vi "Numeric Speed to Formatted String.vi"(8 "error in (no error)":errorcluster, 9 "Speed Units":T1, 10 "Speed":dbl format="%.2f", 11 "ESM303 in":refnum<class "ESM303.lvclass">) -> (0 "error out":errorcluster, 2 "Formatted Speed String":string, 3 "ESM303 out":refnum<class "ESM303.lvclass">)   [LabVIEW 2018, in "ESM303.lvlib" / "ESM303.lvclass"]
uses:
  ESM303.lvclass
  builds/Force Test Stand/Force Test Stand/Force Test Stand.lvlibp/Custom Controls/Speed Units.ctl
  builds/Force Test Stand/Force Test Stand/Force Test Stand.lvlibp/Force Test Stand.lvclass
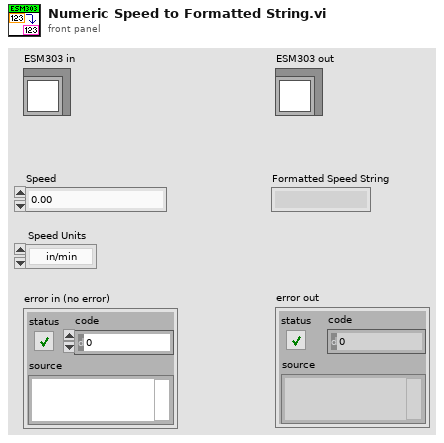
[diagram p1: front panel]
types:
  T1 = typedef "Force Test Stand.lvlibp/Force Test Stand.lvclass/Speed Units.ctl" = enum16{"in/min", "mm/min"}
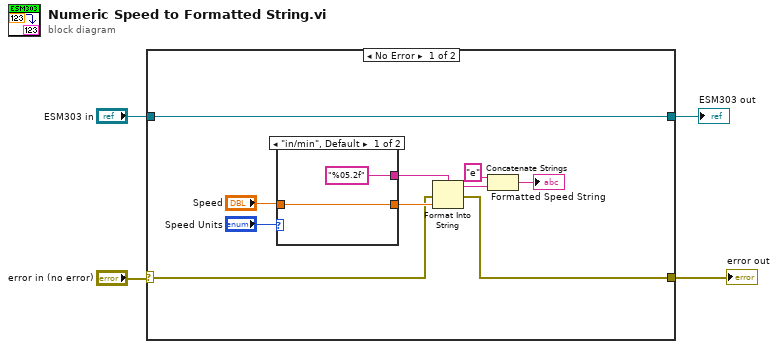
[diagram p0: block diagram]
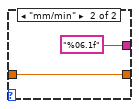
[diagram p2: hidden frame]
diagram:
  n1 = case shown="No Error" "error in (no error)" {
    selector: "error in (no error)" -> [w8 w19]
    tunnel: [w10 w20] -> w4
    tunnel: "ESM303 in" -> [w10 w20]
    tunnel: [w7 w19] -> w1
    frame No Error {
      n2 = case shown="\"in/min\", Default" "Speed Units" {
        tunnel: "Speed" -> [w16 w17]
        tunnel: ["%05.2f" ("format string") "%06.1f" ("format string")] -> w12
        tunnel: [w16 w17] -> w13
        frame "in/min", Default {
        }
        frame "mm/min" {
        }
      }
      n3 = Format Into String(format string=w12, error in=w8, w13) -> (resulting string=w14:string, error out=w7:errorcluster)  [unwired: 1 in]
      n4 = Concatenate Strings("e", w14) -> (→"Formatted Speed String":string)
    }
    frame Error {
    }
  }
  "error out" <- w1
  "ESM303 out" <- w4
